vi "Rename.vi"(6 "Defer restart? (false)":bool, 8 "error in (no error)":errorcluster, 10 "New name":string, 11 "RT Management in":refnum<class "RT Management.lvclass">) -> (0 "error out":errorcluster, 3 "RT Management out":refnum<class "RT Management.lvclass">)   [LabVIEW 2015, in "RT Management.lvlib" / "RT Management.lvclass"]
doc: "Gives an RT target a new hostname, reboots the target, and then returns the new IP address."
uses:
  RT Management.lvclass
  RT Management.lvclass/RT Management.ctl
  Get SysCfg Session.vi
  <resource>/objmgr/nisysapi.rc
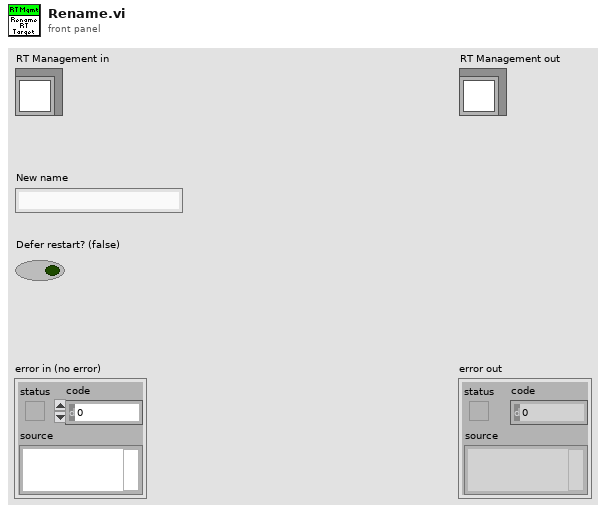
[diagram p1: front panel]
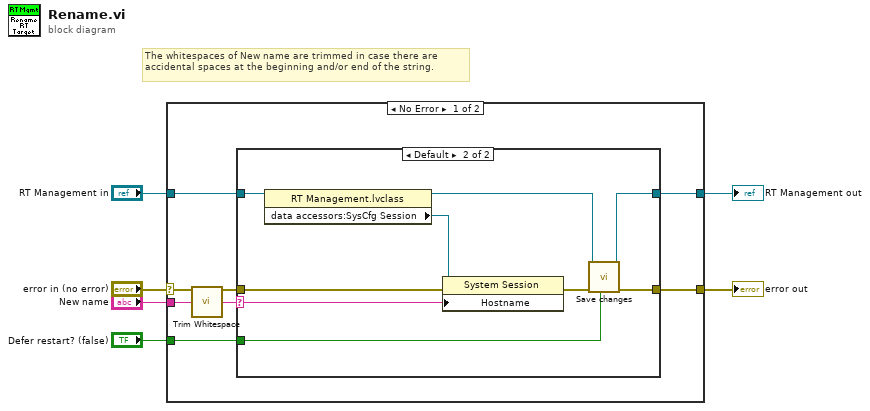
[diagram p0: block diagram]
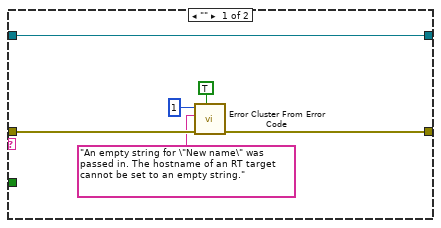
[diagram p2: hidden frame]
diagram:
  # "The whitespaces of New name are trimmed in case there are accidental spaces at the beginning and/or end of the string."
  n1 = case shown="No Error" "error in (no error)" {
    selector: "error in (no error)" -> [w11 w30]
    tunnel: [w13 w30] -> w5
    tunnel: [w10 w29] -> w3
    tunnel: "RT Management in" -> [w12 w29]
    tunnel: "New name" -> [w9 _]
    tunnel: "Defer restart? (false)" -> [w7 _]
    frame No Error {
      n2 = call <vilib>:"Trim Whitespace.vi"("string"=w9) -> ("trimmed string"=w8:string)  [unwired: 1 in]
      n3 = case shown="Default" w8 {
        selector: w8 -> [_ w25]
        tunnel: [w18 w21] -> w13
        tunnel: w12 -> [w19 w28]
        tunnel: w11 -> [w17 w26]
        tunnel: [w19 w22] -> w10
        tunnel: w7 -> [_ w20]
        frame "" {
          n4 = call <vilib>:"Error Cluster From Error Code.vi"("show call chain? (False)"=TRUE, "error in (no error)"=w17, "error message (\"\")"="An empty string for \"New name\" was passed in. The hostname of an RT target cannot be set to an empty string." ("error message (\"\")"), "error code (0)"=1) -> ("error out"=w18:errorcluster)  [unwired: 5 in]
        }
        frame Default {
          n5 = property class="RT Management.lvclass"(reference=w28) -> (reference out=w23:refnum<class "RT Management.lvclass">, "data accessors:SysCfg Session"=w27:refnum<k21>)  [unwired: 1 in, 1 out]
          n6 = property class="System Session"(reference=w27, error in=w26, "Hostname"=w25) -> (error out=w24:errorcluster)  [unwired: 1 out]
          n7 = call "Save changes.vi"("Defer restart? (true)"=w20, "error in (no error)"=w24, "RT Management in"=w23) -> ("error out"=w21:errorcluster, "RT Management out"=w22:refnum<class "RT Management.lvclass">)  [unwired: 7 in]
        }
      }
    }
    frame Error {
    }
  }
  "error out" <- w5
  "RT Management out" <- w3
